vi "AlmacenarDatos.vi"(8 "Nombre del archivo txt":string, 9 "StampTime":string, 10 "Fare.":string, 11 "Cent":string) -> (0 "error out":errorcluster, 2 "all rows":string[][](array[string]))   [LabVIEW 2019]
doc: "Crea una caperta en la ruta de directorio, en esta se crea un archivo de texto creado por el usuario. Posteriormente, se guardarán en este archivo de texto los parámetros de entrada por columnas."
uses:
  <vilib>/Utility/file.llb/Read Delimited Spreadsheet (string).vi
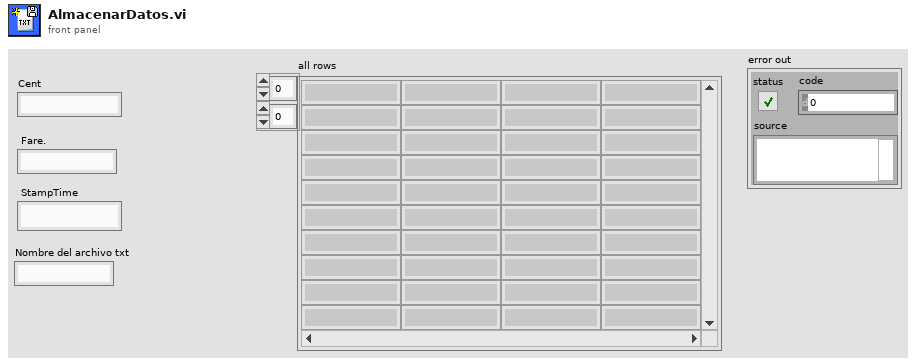
[diagram p1: front panel]
types:
  T1 = enum16{"open", "replace", "create", "open or create", "replace or create", "replace or create with confirmation"}
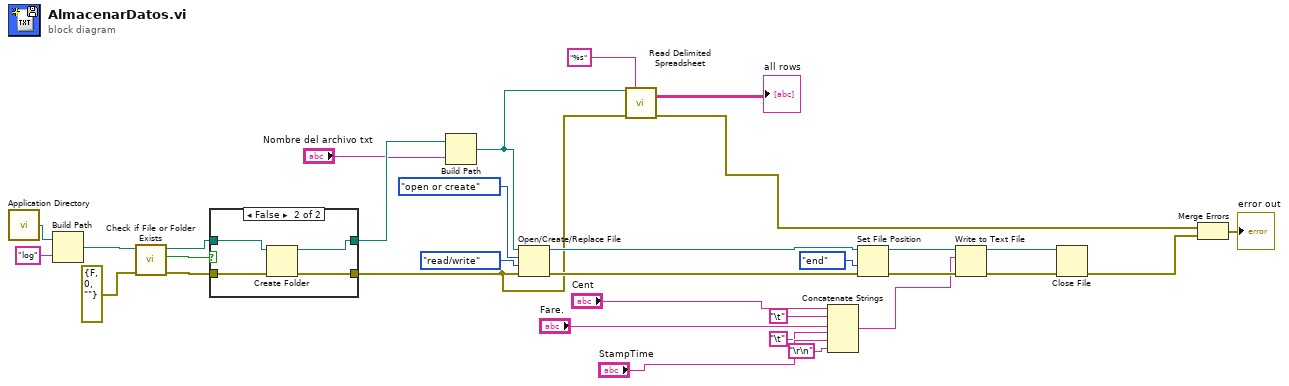
[diagram p0: block diagram]
diagram:
  n1 = call <vilib>:"Application Directory.vi"() -> ("Application Directory"=w13:path)
  n2 = Build Path(base path=w13, name or relative path="log") -> (appended path=w20:path)
  n3 = call <vilib>:"Check if File or Folder Exists.vi"("error in (no error)"=errorcluster {"status"=FALSE, "code"=0, "source"=""}, "path"=w20) -> ("error out"=w9:errorcluster, "file or folder exists?"=w21:bool, "dup path"=w10:path)  [unwired: 7 in]
  n4 = case shown="False" w21 {
    tunnel: [w34 w36] -> w4
    tunnel: w10 -> [w33 w38]
    tunnel: w9 -> [w34 w35]
    tunnel: [w33 w37] -> w22
    frame True {
    }
    frame False {
      n5 = Create Folder(path (use dialog)=w38, error in=w35) -> (created path=w37:path, error out=w36:errorcluster)  [unwired: 1 in, 1 out]
    }
  }
  n6 = Build Path(base path=w22, name or relative path="Nombre del archivo txt") -> (appended path=w5:path)
  n7 = Open/Create/Replace File(file path (use dialog)=w5, error in=w4, operation (0:open)=T1."open or create", access (0:read/write)=enum16{"read/write", "read-only", "write-only"}."read/write") -> (refnum out=w23:refnum<file>, error out=w24:errorcluster)  [unwired: 2 in, 1 out]
  n8 = call-poly <vilib>:"Read Delimited Spreadsheet.vi"("file path (dialog if empty)"=w5, "format (%s)"="%s", "error in (no error)"=w4) -> ("all rows"=→"all rows":string[][], "error out"=w3:errorcluster)  [unwired: 7 in, 4 out]
  n9 = Concatenate Strings("Cent", "\t", "Fare.", "\t", "StampTime", "\r\n") -> (w16:string)
  n10 = Set File Position(refnum=w23, from (0:start)=enum16{"start", "end", "current"}."end", error in=w24) -> (refnum out=w18:refnum<file>, error out=w17:errorcluster)  [unwired: 1 in]
  n11 = Write to Text File(file (use dialog)=w18, text=w16, error in=w17) -> (refnum out=w14:refnum<file>, error out=w15:errorcluster)  [unwired: 1 in, 1 out]
  n12 = Close File(refnum=w14, error in=w15) -> (error out=w2:errorcluster)  [unwired: 1 out]
  n13 = Merge Errors(w3, w2) -> (→"error out":errorcluster)
